vi "Read Measurement Scope.vi"(8 "error in":errorcluster, 10 "Scope Model":string, 11 "Module ID":i32=-1) -> (0 "error out":errorcluster)   [LabVIEW 2020, in "Oscilloscope VI.lvlib"]
doc: "Request to Read Measurement from the Oscilloscope object though class methods.\n_____\nCreated using DQMH Event Scripter 6.0.0.122."
uses:
  Oscilloscope VI.lvlib
  Read Measurement Scope Argument--cluster.ctl
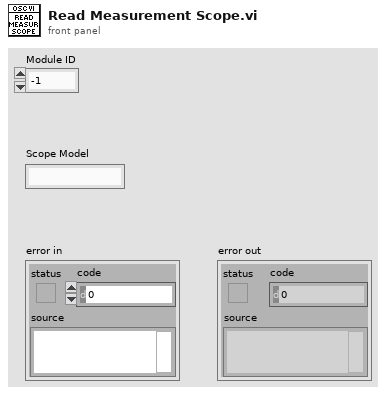
[diagram p1: front panel]
types:
  T1 = typedef "Oscilloscope VI.lvlib/Read Measurement Scope Argument--cluster.ctl" = cluster{"Module ID":i32, "Scope Model":string}
  T2 = typedef "Oscilloscope VI.lvlib/Request Events--cluster.ctl" = cluster{"Stop Module":refnum<user-event>, "Show Panel":refnum<user-event>, "Hide Panel":refnum<user-event>, "Show Diagram":refnum<user-event>, "Get Module Execution Status":refnum<user-event>, "Set Port":refnum<user-event>, "Initialize Scope":refnum<user-event>, "Close Scope":refnum<user-event>, "Autosetup Scope":refnum<user-event>, "Configure Channel Scope":refnum<user-event>, "Read Measurement Scope":refnum<user-event>, "Read Measurement 2 Channels Scope":refnum<user-event>, "Read Waveform Scope":refnum<user-event>, "Reset Scope":refnum<user-event>}
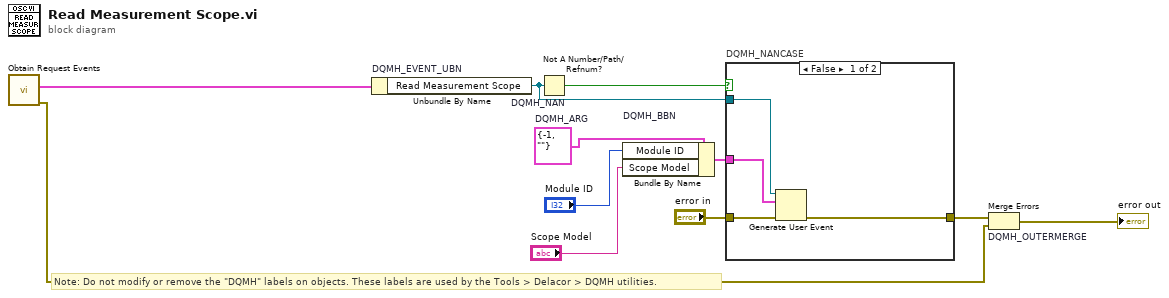
[diagram p0: block diagram]
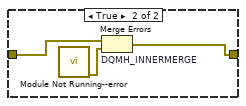
[diagram p2: hidden frame]
diagram:
  w5 = T1 {"Module ID"=-1, "Scope Model"=""}  # DQMH_ARG
  # "Note: Do not modify or remove the \"DQMH\" labels on objects. These labels are used by the Tools > Delacor > DQMH utilities."
  n1 = call "Obtain Request Events.vi"() -> ("error out"=w2:errorcluster, "Oscilloscope VI Request Events"=w1:T2)  [unwired: 10 in]
  n2 = Unbundle By Name "DQMH_EVENT_UBN"(w1) -> ("Read Measurement Scope"=w7:refnum<user-event>)
  n3 = Not A Number/Path/Refnum? "DQMH_NAN"(number/path/refnum=w7) -> (NaN/Path/Refnum?=w8:bool)
  n4 = Bundle By Name "DQMH_BBN"(cluster=w5, "Module ID"="Module ID", "Scope Model"="Scope Model") -> (w9:T1)
  n5 = case "DQMH_NANCASE" shown="False" w8 {
    tunnel: "error in" -> [w15 w18]
    tunnel: [w14 w17] -> w6
    tunnel: w7 -> [w13 _]
    tunnel: w9 -> [w12 _]
    frame False {
      n6 = Generate User Event(user event=w13, event data cluster=w12, error in=w15) -> (error out=w14:errorcluster)  [unwired: 1 in, 1 out]
    }
    frame True {
      n7 = call "Module Not Running--error.vi"() -> ("error out"=w16:errorcluster)  [unwired: 11 in]
      n8 = Merge Errors "DQMH_INNERMERGE"(w18, w16) -> (w17:errorcluster)
    }
  }
  n9 = Merge Errors "DQMH_OUTERMERGE"(w6, w2) -> (→"error out":errorcluster)
